vi "Add VI Documentation.vi"(6 "Method Name":string, 9 "Class Name":string, 10 "URL Format":string, 11 "VI (Struct or Method)":refnum<vi>) -> (3 "VI Dup":refnum<vi>)   [LabVIEW 2014]
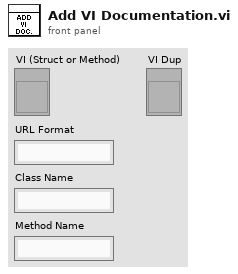
[diagram p1: front panel]
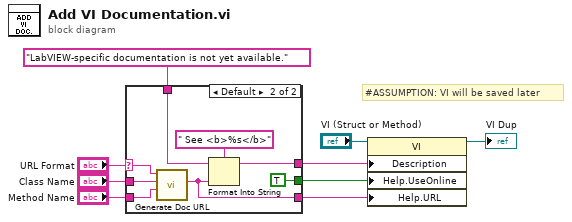
[diagram p0: block diagram]
diagram:
  # "#ASSUMPTION: VI will be saved later"
  n1 = case shown="Default" "URL Format" {
    selector: "URL Format" -> [_ w15]
    tunnel: "LabVIEW-specific documentation is not yet available." -> [w10 w18]
    tunnel: [w10 w17] -> w8
    tunnel: "Class Name" -> [_ w14]
    tunnel: "Method Name" -> [_ w13]
    tunnel: [_ w12] -> w2
    tunnel: [_ TRUE ("Help:Use Web URL")] -> w1
    frame "" {
      # "No URL format specified"
    }
    frame Default {
      n2 = call "Generate Doc URL.vi"("Method Name"=w13, "Owning Entity Name"=w14, "URL Format"=w15) -> ("Final URL"=w12:string)  [unwired: 8 in]
      n3 = Format Into String(format string=" See <b>%s</b>", initial string=w18, w12) -> (resulting string=w17:string)  [unwired: 1 in, 1 out]
    }
  }
  n4 = property class="VI"(reference="VI (Struct or Method)", "Description"=w8, "Help.UseOnline"=w1, "Help.URL"=w2) -> (reference out=→"VI Dup":refnum<vi>)  [unwired: 1 in, 1 out]
